vi "PH_Beamline.Calc Compressor State.vi"(0 "i ref in":refnum<vi>, 2 "PA Exit closed or shining into LL":bool, 3 "Not shining Experiment LB":bool, 5 "error in (no error)":errorcluster) -> (14 "i ref out":refnum<vi>, 19 "error out":errorcluster)   [LabVIEW 2014, in "PH_Beamline.lvlib"]
doc: "This VI calculates the Compresor state of the Beamline."
uses:
  PH_Beamline.lvlib
  PH_SystemInformation/PH_SystemInformationEnabling State.ctl
  PH_Common/PH_Common.lvlib
  PH_SystemInformation/PH_SystemInformation.lvlib
  PH_BL-Master/PH_BL-Master.lvlib
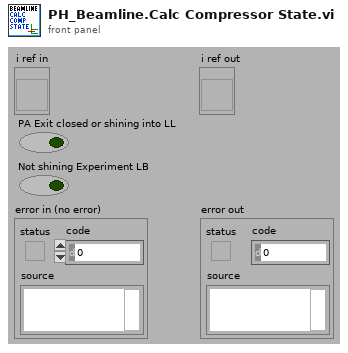
[diagram p1: front panel]
types:
  T1 = typedef "PH_Beamline.lvlib/PH_Beamline.i attribute.ctl" = cluster{"GUI Refs":cluster{"PA ok":refnum<vi>, "MA ok":refnum<vi>, "fs FE ok":refnum<vi>, "ns FE ok":refnum<vi>, "PA ED ok":refnum<vi>, "MAS ok":refnum<vi>, "Booster ok":refnum<vi>, "Mirrortower ok":refnum<vi>, "In.-Box ok":refnum<vi>, "Compressor ok":refnum<vi>, "Experiment LB ok":refnum<vi>, "Experiment LL ok":refnum<vi>, "PHELIX_Beckhoff_Watchdog":refnum<vi>, "Shutters closed":refnum<vi>, "uOPA ok":refnum<vi>, "Vacuum no shotcond Comp LB":refnum<vi>}, "Refs BL MA":refnum<vi>[], "Refs BL MA-IB":refnum<vi>[], "Refs BL fs":refnum<vi>[], "Refs BL PA ED":refnum<vi>[], "Refs BL MAS":refnum<vi>[], "Refs BL Boo":refnum<vi>[], "Refs BL ns":refnum<vi>[], "Refs BL Mirrortower":refnum<vi>[], "Refs BL Compressor":refnum<vi>[], "Refs BL Exp LB":refnum<vi>[], "Radiation Safety":cluster{"Exp Laserbay":cluster{"Ref Op Mode":refnum<vi>, "Ref Laserbay evacuated":refnum<vi>, "Tagname LB evacuated":string, "Shot Mode":T2, "Laserbay evacuated?":i32, "Tagname HV room locked":string, "HV room locked?":i32, "Ref HV room locked":refnum<vi>, "Tagname bridged?":string, "Ref Bridge":refnum<vi>, "I<1E18W/cm²":bool}, "Exp Laserlab":cluster{"Ref Op Mode":refnum<vi>, "Ref Laserlab evacuated":refnum<vi>, "Tagname LL evacuated":string, "Shot Mode":T2, "Laserlab evacuated?":i32, "Tagname bridged?":string, "Ref Bridge":refnum<vi>, "I<1E18W/cm²":bool}}, "Refs BL LL":refnum<vi>[], "PP Igni Heating GUI Refs":refnum<vi>[], "PP Igni Heating Tagnames ":string[], "Refs BL PA":cluster{"undelayed Line before Shutter":refnum<vi>[], "undelayed Line after Shutter":refnum<vi>[], "before Bypass":refnum<vi>[], "delayed Line before Shutter":refnum<vi>[], "delayed Line after Shutter":refnum<vi>[], "before Shutter Input":refnum<vi>[], "after Shutter Input":refnum<vi>[], "Bypass":refnum<vi>[], "before Shutter Exit":refnum<vi>[], "after Shutter Exit":refnum<vi>[], "to MA":refnum<vi>[], "to Lab":refnum<vi>[]}, "BL":cluster{"YLF_BL_Status":i32, "fs_BL_Status":i32, "fs_YLF_BL_Status":i32, "ns_BL_Status":i32, "PA_Input_BL_Status":i32, "PA_UnDelay_BL_Status":i32, "PA_Delay_BL_Status":i32, "PA_BL_Status":i32, "PA_Bypass_BL_Status":i32, "PA_Exit_BL_Status":i32, "PA_LL_BL_Status":i32, "LL_BL_Status":i32, "PA_MA_BL_Status":i32, "MA_Exit_BL_Status":i32, "MA_Z6_BL_Status":i32, "Z6_BL_Status":i32, "MA_LB_BL_Status":i32, "LB_TB2_BL_Status":i32, "PA_before_Bypass_BL_Status":i32, "LB_TB3_BL_Status":i32}, "State Subsystems":cluster{"PA":bool, "MA":bool, "ns FE":bool, "fs FE":bool, "PA ED":bool, "In.-Box":bool, "MAS":bool, "Booster":bool, "Mirrortower":bool, "Compressor":bool, "Experiment LB":bool, "Experiment LL":bool, "uOPA":bool}, "Status Subscriber Information":T3, "Refs BL uOPA":refnum<vi>[], "PA_Input_2_Beam_6PWpGUI not linked?":bool, "PA_Input_Delay_6PGUI not linked?":bool, "Settings":T6}
  T2 = typedef "PH_Beamline.lvlib/PH_Beamline.Operation Mode.ctl" = i32
  T3 = typedef "PH_Beamline.lvlib/PH_Beamline.Status Subscriber Information.ctl" = cluster{"fs Swich YLF":T4, "fs Exit Shutter":T4, "ns Exit Shutter":T4, "PA Input Shutter":T4, "PA PC WP":T4, "PA PC WP 2":T4, "PA Bypass In":T4, "PA Bypass Out":T4, "PA CH 1":T4, "PA delayed":T4, "PA non delayed":T4, "PA Exit Shutter":T4, "PA Switch Lab":T4, "PA Bridge CH Input MA":T4, "MA Diffusor IB":T4, "MA IB Ready":T4, "MA CH 1":T4, "MA CH 2":T4, "MA CH 3":T4, "MA CH 4":T4, "MA Shutter Align Cam":T4, "MA Position MM5":T4, "Calorimeter Switch":T4, "BL Z6 CH 9":T4, "BL Z6 Beamdump":T4, "BL Z6 Shutter":T4, "COS Sensitivity Switch":T4, "Exp LB Shutter":T4, "Exp LB TB 2":T4, "Exp LB TB 3":T4, "PA LL Input CH":T4, "PA LL Output CH":T4, "LL Comp Input Shutter":T4, "LL Comp Output Shutter":T4, "LL Comp FF Shutter":T4, "Exp LL Shutter":T4, "MA IM In IB":T4, "MA IM Out IB":T4, "MA DB In IB":T4, "MA DB Out IB":T4, "Exp LB Shutter Interlock":T4, "Exp LL Shutter Interlock":T4, "MM1 Force Sensor":T4}
  T4 = typedef "PH_BL-Master.lvlib/PH_BL-Master.Status Subscriber Information.ctl" = cluster{"Index of element":i32, "Attributeset":T5}
  T5 = typedef "PH_BL-Master.lvlib/PH_BL-Master.Attribute Set.ctl" = enum16{"Boolean Status Service Subscriber", "Picture Status Service Subscriber"}
  T6 = typedef "PH_Beamline_Chief.lvlib/PH_Beamline_Chief.Settings.ctl" = cluster{"PA Doublepass Mode":bool, "Compressor Vaccuum LB not relevant":bool, "Windowshutter TB2 not relevant":bool, "Windowshutter TB3 not relevant":bool}
  T7 = enum16{"All, Default", "PreAmp", "MainAmp", "Compressor", "Experiment", "Z6 Telescope"}
  T8 = enum16{"Laser", "PreAmp", "MainAmp", "Exp 1", "Exp 2", "Exp 3", "Exp 4"}[]
  T9 = typedef "PH_SystemInformation.lvlib/PH_SystemInformationEnabling State.ctl" = i32
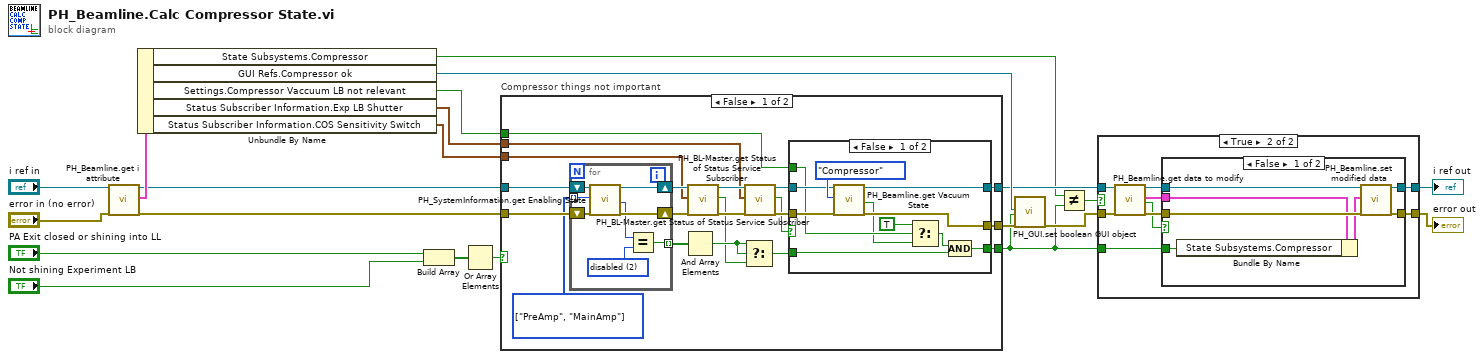
[diagram p0: block diagram]
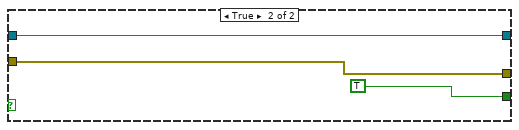
[diagram p5: hidden frame]
diagram:
  n1 = call "PH_Beamline.get i attribute.vi"("i ref in"="i ref in", "error in (no error)"="error in (no error)") -> ("i ref out"=w5:refnum<vi>, "i attribute"=w18:T1, "error out"=w4:errorcluster)  [unwired: 15 in]
  n2 = Unbundle By Name(w18) -> ("State Subsystems.Compressor"=w11:bool, "GUI Refs.Compressor ok"=w19:refnum<vi>, "Settings.Compressor Vaccuum LB not relevant"=w1:bool, "Status Subscriber Information.Exp LB Shutter"=w3:T4, "Status Subscriber Information.COS Sensitivity Switch"=w2:T4)
  n3 = Build Array("PA Exit closed or shining into LL", "Not shining Experiment LB") -> (w17:bool[])
  n4 = Or Array Elements(Boolean array=w17) -> (logical OR=w21:bool)
  n5 = case "Compressor things not important" shown="False" w21 {
    tunnel: w5 -> [w33 w66]
    tunnel: [w40 w66] -> w15
    tunnel: w4 -> [w31 w65]
    tunnel: [w41 w65] -> w20
    tunnel: [w39 TRUE] -> w10
    tunnel: w3 -> [w24 _]
    tunnel: w2 -> [w23 _]
    tunnel: w1 -> [w22 _]
    frame False {
      w29 = T8 [enum."PreAmp", enum."MainAmp"] items=["Laser", "PreAmp", "MainAmp", "Exp 1", "Exp 2", "Exp 3", "Exp 4"]
      n6 = for {
        shift-right: [w48] -> w32
        shift-left: w33 -> [w49]
        shift-right: [w46] -> w30
        shift-left: w31 -> [w47]
        tunnel: w29 -> [w45] mode=indexing
        tunnel: [w42] -> w28 mode=indexing
        w43 = T9 2 items=["no info", "not disabled", "disabled"] ("y")
        n7 = call "PH_SystemInformation.get Enabling State.vi"("i ref in"=w49, "Wanted State"=w45, "error in (no error)"=w47) -> ("i ref out"=w48:refnum<vi>, "Enabling State"=w44:T9, "error out"=w46:errorcluster)  [unwired: 14 in]
        n8 = Equal?(x=w44, y=w43) -> (x = y?=w42:bool)
      }
      n9 = And Array Elements(Boolean array=w28) -> (logical AND=w27:bool)
      n10 = call "PH_BL-Master.get Status of Status Service Subscriber.vi"("i ref in"=w32, "Wanted Status Subscriber Information"=w23, "error in (no error)"=w30) -> ("i ref out"=w36:refnum<vi>, "on/true/in?"=w26:bool, "error out"=w38:errorcluster)  [unwired: 11 in, 3 out]
      n11 = Select(t=w27, s=w27, f=w26) -> (s? t:f=w25:bool)
      n12 = call "PH_BL-Master.get Status of Status Service Subscriber.vi"("i ref in"=w36, "Wanted Status Subscriber Information"=w24, "error in (no error)"=w38) -> ("i ref out"=w35:refnum<vi>, "on/true/in?"=w34:bool, "error out"=w37:errorcluster)  [unwired: 11 in, 3 out]
      n13 = case shown="False" w34 {
        tunnel: [w60 w62] -> w41
        tunnel: [w59 w63] -> w40
        tunnel: w25 -> [w57 w61]
        tunnel: [w56 w61] -> w39
        tunnel: w37 -> [w53 w62]
        tunnel: w35 -> [w54 w63]
        tunnel: w22 -> [w52 _]
        frame False {
          n14 = call "PH_Beamline.get Vacuum State.vi"("i ref in"=w54, "Subsystem"=T7."Compressor", "error in (no error)"=w53) -> ("i ref out"=w59:refnum<vi>, "vacua in range"=w51:bool, "error out"=w60:errorcluster)  [unwired: 14 in]
          n15 = Select(t=TRUE ("f"), s=w52, f=w51) -> (s? t:f=w55:bool)
          n16 = Compound Arithmetic op=AND(w55, w57) -> (w56:bool)
        }
        frame True {
        }
      }
    }
    frame True {
    }
  }
  n17 = call "PH_GUI.set boolean GUI object.vi"("Boolean Knob GUI Ref"=w19, "Value"=w10, "error in (no error)"=w20) -> ("error out"=w13:errorcluster)  [unwired: 16 in]
  n18 = Not Equal?(x=w11, y=w10) -> (x != y?=w16:bool)
  n19 = case shown="True" w16 {
    tunnel: [w68 w73] -> w14
    tunnel: [w67 w72] -> w12
    tunnel: w10 -> [_ w71]
    tunnel: w13 -> [w67 w70]
    tunnel: w15 -> [w68 w69]
    frame False {
    }
    frame True {
      n20 = call "PH_Beamline.get data to modify.vi"("i ref in"=w69, "error in (no error)"=w70) -> ("i ref out"=w76:refnum<vi>, "i attribute"=w74:T1, "timed out"=w75:bool, "error out"=w77:errorcluster)  [unwired: 14 in]
      n21 = case shown="False" w75 {
        tunnel: w77 -> [w84 w85]
        tunnel: w76 -> [w83 w86]
        tunnel: [w82 w85] -> w72
        tunnel: [w81 w86] -> w73
        tunnel: w74 -> [w80 _]
        tunnel: w71 -> [w78 _]
        frame False {
          n22 = Bundle By Name(cluster=w80, "State Subsystems.Compressor"=w78) -> (w79:T1)
          n23 = call "PH_Beamline.set modified data.vi"("i ref in"=w83, "i attribute"=w79, "error in (no error)"=w84) -> ("i ref out"=w81:refnum<vi>, "error out"=w82:errorcluster)  [unwired: 15 in]
        }
        frame True {
        }
      }
    }
  }
  "i ref out" <- w14
  "error out" <- w12
